vi "Convert Data From Database to QDFunction.vi"(8 "error in (no error)":errorcluster, 10 "FetchedData":variant[](array[variant]), 11 "NormalQDFunc in":refnum<class "NormalQDFunc.lvclass">) -> (0 "error out":errorcluster, 3 "NormalQDFunc out":refnum<class "NormalQDFunc.lvclass">)   [LabVIEW 2015, in "NormalQDFunc.lvclass"]
uses:
  NormalQDFunc.lvclass
  NormalQDFunc.lvclass/NormalQDFunc.ctl
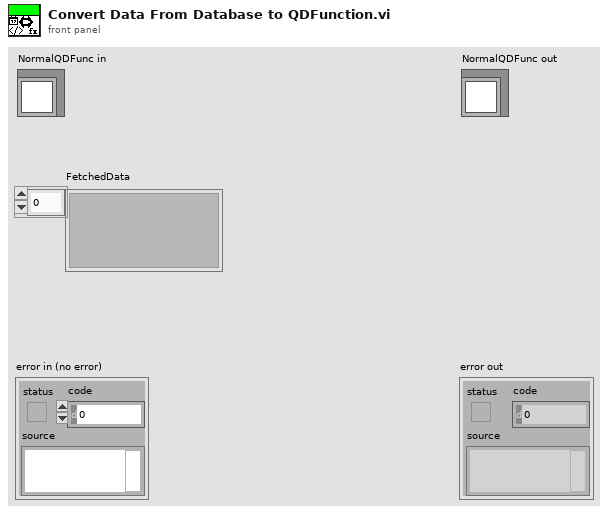
[diagram p1: front panel]
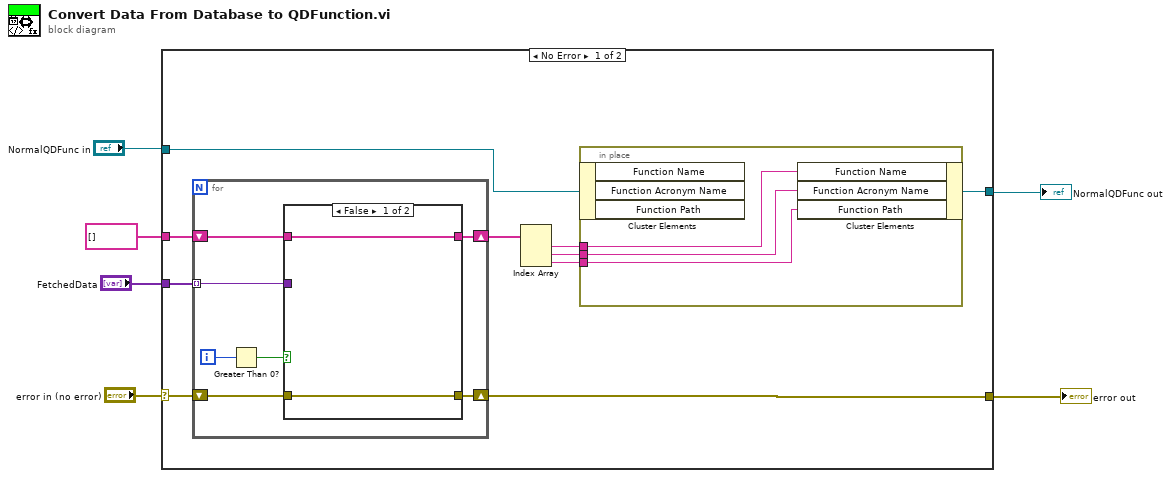
[diagram p0: block diagram]
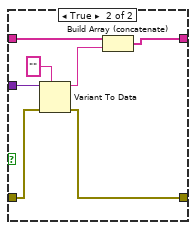
[diagram p2: hidden frame]
diagram:
  n1 = case shown="No Error" "error in (no error)" {
    selector: "error in (no error)" -> [w15 w37]
    tunnel: "FetchedData" -> [w16 _]
    tunnel: string[] [] -> [w14 _]
    tunnel: [w13 w37] -> w3
    tunnel: "NormalQDFunc in" -> [w11 w36]
    tunnel: [w7 w36] -> w1
    frame No Error {
      n2 = for {
        tunnel: w16 -> [w24] mode=indexing
        shift-right: [w21] -> w13
        shift-left: w15 -> [w23]
        shift-right: [w20] -> w12
        shift-left: w14 -> [w22]
        i -> [w26]
        n3 = Greater Than 0?(x=w26) -> (x > 0?=w25:bool)
        n4 = case shown="False" w25 {
          tunnel: w24 -> [_ w35]
          tunnel: w23 -> [w27 w33]
          tunnel: w22 -> [w28 w32]
          tunnel: [w27 w30] -> w21
          tunnel: [w28 w29] -> w20
          frame False {
          }
          frame True {
            n5 = Variant To Data(error in=w33, type="", Variant=w35) -> (data=w31:string, error out=w30:errorcluster)
            n6 = Build Array (concatenate)(w32, w31) -> (w29:string[])
          }
        }
      }
      n7 = Index Array(array=w12) -> (element #1=w10:string, element #2=w9:string, element #3=w8:string)  [unwired: 3 in]
      n8 = in-place {
        in-place-border: w10 -> [w19]
        in-place-border: w9 -> [w18]
        in-place-border: w8 -> [w17]
        n9 = in-place-cluster #1(w11) -> ()  [unwired: 3 out]
        n10 = in-place-cluster #1("Function Name"=w19, "Function Acronym Name"=w18, "Function Path"=w17) -> (w7:refnum<class "NormalQDFunc.lvclass">)
      }
    }
    frame Error {
    }
  }
  "error out" <- w3
  "NormalQDFunc out" <- w1
